vi "Initial Values-Unbundler-DBL.vi"(8 "error in (no error)":errorcluster, 9 "Keys Array":T2, 10 "Section name":string, 11 "User profile ini file ref":T1) -> (0 "error out":errorcluster, 3 "User profile ini file ref":T1)   [LabVIEW 2013]
uses:
  Typedefs/Ini file interface (DBL).ctl
  <vilib>/Utility/config.llb/Config Data RefNum.ctl
  User Interface/Visualisation/Functional Imaging Viewer/Typedefs/Get-Set-Clear Control.ctl
  User Interface/Visualisation/Timelapse Viewer/Globals/gl_Time series viewer globals.vi
  Global Variables/gl_UI Ctrl Refs.vi
  <vilib>/Utility/config.llb/NI_LVConfig.lvlib
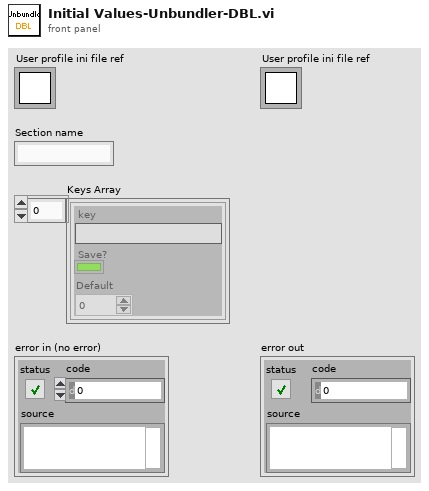
[diagram p1: front panel]
types:
  T1 = typedef "NI_LVConfig.lvlib/Config Data RefNum.ctl" = refnum<k1>
  T2 = typedef "Ini file interface (DBL).ctl" = cluster{"key":string, "Save?":bool, "Default":dbl}[]
  T3 = typedef "Get-Set-Clear Control.ctl" = enum16{"Get", "Set", "Clear"}
  T4 = typedef "UI ctrl refs cluster.ctl" = cluster{"Top level VI path":path, "Top level VI ref":refnum<vi>, "User menu ref":refnum<k9>, "Sub Panel control":refnum<vi>, "Imaging Param Tab":refnum<vi>, "Occurrence-Start drivers":refnum<k4>, "Occurrence-Speed logging initialised":refnum<k4>, "Occurrence-XYZ stage initialised":refnum<k4>, "Exit button":refnum<vi>, "Status ind":refnum<vi>, "Return to Origin":refnum<vi>, "Speed Logging":refnum<vi>, "Time Lapse":refnum<vi>, "Live Imaging":refnum<vi>, "AOL Z Stack":refnum<vi>, "Motor Z Stack":refnum<vi>, "Funct Acq button":refnum<vi>, "Hard Shutter":refnum<vi>, "Virtual Shutter":refnum<vi>, "Laser Power":refnum<vi>, "AOL Mode":refnum<vi>, "Frame Size":refnum<vi>, "Field of View":refnum<vi>, "Dwell Time":refnum<vi>, "Zoom":refnum<vi>, "AOL Z":refnum<vi>, "Objective":refnum<vi>, "Axis":refnum<vi>, "Paths & Names":refnum<vi>, "Experiment folder path (ind.)":refnum<vi>, "Last State (Ind.)":refnum<vi>, "Laser wavelength ind (nm)":refnum<vi>, "Averages":refnum<vi>, "Angle (degrees)":refnum<vi>, "X centre":refnum<vi>, "Y centre":refnum<vi>, "Plane Mode":refnum<vi>, "# Planes":refnum<vi>, "Z Start":refnum<vi>, "Z Stop":refnum<vi>, "Z Step":refnum<vi>, "PMT 1":refnum<vi>, "PMT 2":refnum<vi>, "Stage XYZ Position":refnum<vi>, "Pockels@Z Start":refnum<vi>, "Pockels@Z Stop":refnum<vi>, "Obtain Z Start":refnum<vi>, "Obtain Z Stop":refnum<vi>, "Live stim.trig.period":refnum<vi>, "Live stim.trig.enable":refnum<vi>, "Funct. Acq. Pockels Modulation":refnum<vi>, "Enable Video Recording":refnum<vi>, "Video Record-Live Imaging":refnum<vi>, "Video Record-Funct acq":refnum<vi>, "AOL Z-stack Chirps Ready (ind)":refnum<vi>, "Center freq ind (nm)":refnum<vi>, "Logging queue (ind)":refnum<vi>, "Back aperture power (ind.)":refnum<vi>, "Power after objective (ind.)":refnum<vi>, "Switch user":refnum<vi>}
  T5 = typedef "AOL_Globals.ctl" = cluster{"Imaging Protocol":T6, "Number of POI":u16, "Number of Miniscans":u16, "Number of Trials":u16, "Number of Cycles ":u64, "# Averaged Frames":u16, "Laser power (%)":u8, "Pockels":dbl, "Acquisition Length (sec)":dbl, "Fill time (us)":dbl, "POI Dwell time (us)":dbl, "Miniscan Dwell time per pixel (us)":dbl, "PMT 1":dbl, "PMT 2":dbl, "Back Apperture":dbl, "Frame Size":T7, "Center Frequency":dbl, "Field of View":dbl, "DwellTime (us)":dbl, "Wavelength (nm)":dbl, "Zoom":dbl, "AOL Z":dbl, "AOL Mode":T8, "GridXY":dbl, "GridZ":dbl, "TriggerPeriod (sec)":dbl, "Number of Pixels in Miniscan":u16, "Experiment folder path":path, "X centre":dbl, "Y centre":dbl, "Angle (degrees)":dbl, "Plane Mode":T9, "Threshold":u16[], "Regenerate Chirps":bool, "Rectangle ROI length (pixels)":u16, "Rectangle ROI height (pixels)":u16, "AOD fill":u16, "Samples Wait after Trigger":u16, "StartUp Delay":i32, "Slip Cycle":u32, "Add Cycle":bool}
  T6 = typedef "Imaging Protocols enum.ctl" = enum16{"AOL Z-Stack", "Motor Z Stack", "Functional Acquisition", "Single Plane Acquisition", "Volume Acquisition", "Live Imaging", "Live Plane Imaging", "Live Volume Imaging"}
  T7 = typedef "Frame Size.ctl" = u16
  T8 = typedef "AOL modes.ctl" = enum16{"Raster", "Structural", "Pointing", "Mini Scan", "Alignment"}
  T9 = typedef "Plane Mode.ctl" = u16
  T10 = typedef "Stitch layout spec cluster.ctl" = cluster{"Timelapse image":cluster{"Image position":T11}, "Cam 1":cluster{"Image position":T11}, "Cam 2":cluster{"Image position":T11}, "Cam 3":cluster{"Image position":T11}, "Cam 4":cluster{"Image position":T11}}
  T11 = typedef "Image stitching positions.ctl" = enum16{"Top left", "Top right", "Bottom left", "Bottom right", "Not used"}
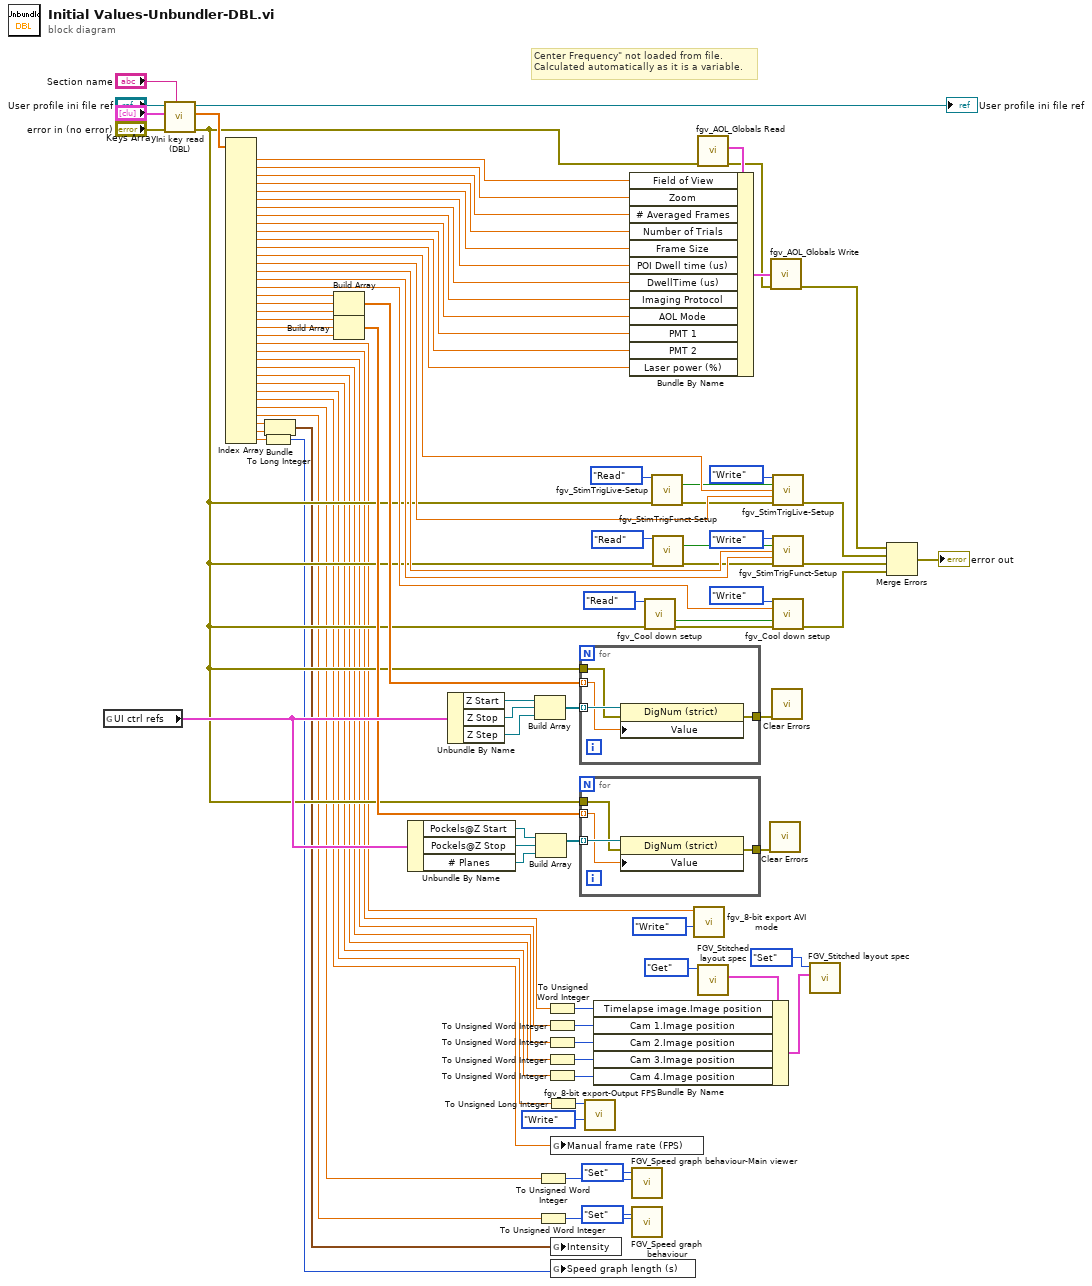
[diagram p0: block diagram]
diagram:
  # "Center Frequency\" not loaded from file.\nCalculated automatically as it is a variable."
  n1 = global read "gl_UI Ctrl Refs.vi" "UI ctrl refs"() -> (w54:T4)
  n2 = call "Ini key read (DBL).vi"("Section name"="Section name", "error in (no error)"="error in (no error)", "Parameter names & setup"="Keys Array", "Ini file refnum in"="User profile ini file ref") -> ("error out"=w37:errorcluster, "Value read/used"=w64:dbl[], "Ini file refnum out"=→"User profile ini file ref":T1)  [unwired: 5 in]
  n3 = Index Array(array=w64) -> (element #1=w75:dbl, element #2=w82:dbl, element #3=w83:dbl, element #4=w84:dbl, element #5=w85:dbl, element #6=w86:dbl, element #7=w87:dbl, element #8=w88:dbl, element #9=w89:dbl, element #10=w90:dbl, element #11=w81:dbl, element #12=w80:dbl, element #13=w79:dbl, element #14=w78:dbl, element #15=w77:dbl, element #16=w76:dbl, element #17=w94:dbl, element #18=w52:dbl, element #19=w51:dbl, element #20=w50:dbl, element #21=w48:dbl, element #22=w47:dbl, element #23=w34:dbl, element #24=w21:dbl, element #25=w20:dbl, element #26=w19:dbl, element #27=w18:dbl, element #28=w17:dbl, element #29=w16:dbl, element #30=w15:dbl, element #31=w14:dbl, element #32=w11:dbl, element #33=w10:dbl, element #34=w5:dbl, element #35=w4:dbl, element #36=w2:dbl)  [unwired: 36 in]
  n4 = To Long Integer(number=w2) -> (32bit integer=w1:i32)
  n5 = Bundle("value"=w5, "value"=w4) -> (w3:cluster{"value":dbl, "value":dbl})  [unwired: 1 in]
  n6 = Build Array(w52, w51, w50) -> (w49:dbl[])
  n7 = Build Array(w48, w47, w34) -> (w46:dbl[])
  n8 = Unbundle By Name(w54) -> ("Pockels@Z Start"=w55:refnum<vi>, "Pockels@Z Stop"=w56:refnum<vi>, "# Planes"=w35:refnum<vi>)
  n9 = Unbundle By Name(w54) -> ("Z Start"=w60:refnum<vi>, "Z Stop"=w58:refnum<vi>, "Z Step"=w57:refnum<vi>)
  n10 = Build Array(w60, w58, w57) -> (w59:refnum<vi>[])
  n11 = Build Array(w55, w56, w35) -> (w53:refnum<vi>[])
  n12 = To Unsigned Word Integer(number=w11) -> (unsigned 16bit integer=w7:u16)
  n13 = To Unsigned Word Integer(number=w10) -> (unsigned 16bit integer=w6:u16)
  n14 = To Unsigned Word Integer(number=w20) -> (unsigned 16bit integer=w29:u16)
  n15 = To Unsigned Word Integer(number=w19) -> (unsigned 16bit integer=w28:u16)
  n16 = To Unsigned Word Integer(number=w18) -> (unsigned 16bit integer=w27:u16)
  n17 = To Unsigned Word Integer(number=w17) -> (unsigned 16bit integer=w26:u16)
  n18 = To Unsigned Word Integer(number=w16) -> (unsigned 16bit integer=w25:u16)
  n19 = To Unsigned Long Integer(number=w15) -> (unsigned 32bit integer=w22:u32)
  n20 = global write "gl_Time series viewer globals.vi" "Manual frame rate (FPS)"(w14) -> ()
  n21 = global write "gl_Time series viewer globals.vi" "Intensity"(w3) -> ()
  n22 = global write "gl_Time series viewer globals.vi" "Speed graph length (s)"(w1) -> ()
  n23 = for {
    tunnel: w59 -> [w98] mode=indexing
    tunnel: w49 -> [w97] mode=indexing
    tunnel: [w96] -> w13
    tunnel: w37 -> [w95]
    n24 = property class="DigNum (strict)"(reference=w98, error in=w95, "Value"=w97) -> (error out=w96:errorcluster)  [unwired: 1 out]
  }
  n25 = for {
    tunnel: w53 -> [w102] mode=indexing
    tunnel: w46 -> [w101] mode=indexing
    tunnel: [w100] -> w12
    tunnel: w37 -> [w99]
    n26 = property class="DigNum (strict)"(reference=w102, error in=w99, "Value"=w101) -> (error out=w100:errorcluster)  [unwired: 1 out]
  }
  n27 = call "fgv_8-bit export-Output FPS.vi"("Function"=enum16{"Intialize", "Write", "Read", "Clear"}."Write", "Frames Per Second"=w22) -> ()  [unwired: 8 in, 2 out]
  n28 = call "FGV_Speed graph behaviour-Main viewer.vi"("Function"=Get-Set-Clear_Control."Set", "Speed graph behaviour"=w7) -> ()  [unwired: 8 in, 2 out]
  n29 = call "FGV_Speed graph behaviour.vi"("Function"=Get-Set-Clear_Control."Set", "Speed graph behaviour"=w6) -> ()  [unwired: 8 in, 2 out]
  n30 = call "fgv_Cool down setup.vi"("Function"=enum16{"Intialize", "Write", "Read", "Clear"}."Read", "error in (no error)"=w37) -> ("Enable cool-down time"=w93:bool, "error out"=w40:errorcluster)  [unwired: 11 in, 1 out]
  n31 = call "fgv_StimTrigLive-Setup.vi"("Function"=enum16{"Intialize", "Write", "Read", "Clear"}."Read", "error in (no error)"=w37) -> ("Live stim.trig.enable"=w70:bool, "error out"=w38:errorcluster)  [unwired: 10 in, 2 out]
  n32 = call "fgv_StimTrigFunct-Setup.vi"("Function"=enum16{"Intialize", "Write", "Read", "Clear"}."Read", "error in (no error)"=w37) -> ("Live stim.trig.enable"=w73:bool, "error out"=w39:errorcluster)  [unwired: 10 in, 2 out]
  n33 = call "fgv_8-bit export AVI mode.vi"("Function"=enum16{"Intialize", "Write", "Read", "Clear"}."Write", "AVI mode"=w21) -> ()  [unwired: 8 in, 2 out]
  n34 = call "fgv_AOL_Globals Read.vi"("error in (no error)"=w37) -> ("error out"=w45:errorcluster, "AOL_Globals"=w74:T5)  [unwired: 8 in, 1 out]
  n35 = Bundle By Name(cluster=w74, "Field of View"=w75, "Zoom"=w82, "# Averaged Frames"=w83, "Number of Trials"=w84, "Frame Size"=w85, "POI Dwell time (us)"=w86, "DwellTime (us)"=w87, "Imaging Protocol"=w88, "AOL Mode"=w89, "PMT 1"=w90, "PMT 2"=w81, "Laser power (%)"=w80) -> (w67:T5)
  n36 = call "FGV_Stitched layout spec.vi"("Function"=Get-Set-Clear_Control."Get") -> ("Stitch layout spec"=w31:T10)  [unwired: 9 in, 1 out]
  n37 = Bundle By Name(cluster=w31, "Timelapse image.Image position"=w29, "Cam 1.Image position"=w28, "Cam 2.Image position"=w27, "Cam 3.Image position"=w26, "Cam 4.Image position"=w25) -> (w32:T10)
  n38 = call <vilib>:"Clear Errors.vi"("error in (no error)"=w12) -> ()  [unwired: 6 in, 1 out]
  n39 = call "fgv_AOL_Globals Write.vi"("error in (no error)"=w45, "AOL_Globals"=w67) -> ("error out"=w41:errorcluster)  [unwired: 9 in]
  n40 = call <vilib>:"Clear Errors.vi"("error in (no error)"=w13) -> ()  [unwired: 6 in, 1 out]
  n41 = call "fgv_StimTrigLive-Setup.vi"("Function"=enum16{"Intialize", "Write", "Read", "Clear"}."Write", "Live stim.trig.enable"=w70, "Live stim.trig.period (sec)"=w79, "Live stim.trig.width (ms)"=w78, "error in (no error)"=w38) -> ("error out"=w42:errorcluster)  [unwired: 7 in, 3 out]
  n42 = call "fgv_StimTrigFunct-Setup.vi"("Function"=enum16{"Intialize", "Write", "Read", "Clear"}."Write", "Live stim.trig.enable"=w73, "Funct stim.trig.delay (sec)"=w77, "Funct stim.trig.width (ms)"=w76, "error in (no error)"=w39) -> ("error out"=w43:errorcluster)  [unwired: 7 in, 3 out]
  n43 = call "fgv_Cool down setup.vi"("Function"=enum16{"Intialize", "Write", "Read", "Clear"}."Write", "Cool-down time (s)"=w94, "Enable cool-down time"=w93, "error in (no error)"=w40) -> ("error out"=w44:errorcluster)  [unwired: 9 in, 2 out]
  n44 = call "FGV_Stitched layout spec.vi"("Stitch layout spec"=w32, "Function"=Get-Set-Clear_Control."Set") -> ()  [unwired: 8 in, 2 out]
  n45 = Merge Errors(w41, w42, w43, w44) -> (→"error out":errorcluster)
